vi "Insert.vi"(6 "Item":T1={"Item offset"=0, "Offset past Item"=0, "Name offset"=0, "Offset past Name"=0, "Found"=FALSE, "Item Type"=enum."Parser Error", "Item Index"=-1}, 9 "<JSON>name":string, 10 "JSON to Insert":string, 11 "JSON in":string) -> (1 "Inserted Item Offset":i32, 2 "Found":bool, 3 "string":string)   [LabVIEW 2017, in "JSONtext.lvlib"]
uses:
  JSONtext.lvlib
  Parsing/Found Items.ctl
  Parsing/Parsing State.ctl
  Parsing/Advance past whitespace.vi
  <vilib>/JDP Science/JDP Science Common Utilities/Trim Whitespace__JDP.vi
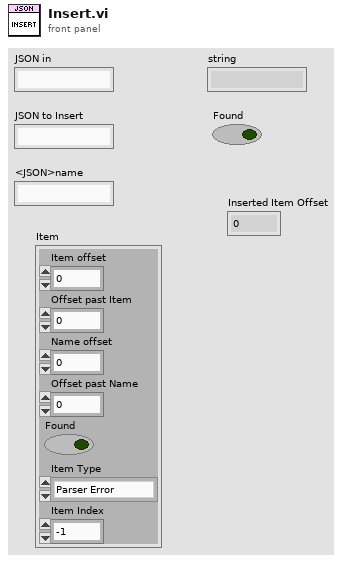
[diagram p1: front panel]
types:
  T1 = typedef "JSONtext.lvlib/Found Items.ctl" = cluster{"Item offset":i32, "Offset past Item":i32, "Name offset":i32, "Offset past Name":i32, "Found":bool, "Item Type":T2, "Item Index":i32}
  T2 = typedef "JSONtext.lvlib/Parsing State.ctl" = enum16{"Parser Error", "Object", "Array", "String", "Number/Other", "Leading Whitespace", "Object end", "Array end", "Value end"}
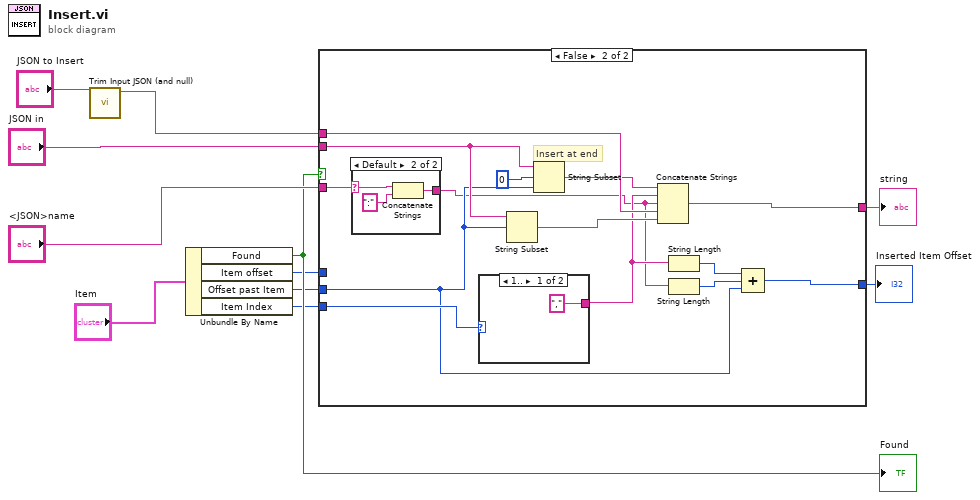
[diagram p0: block diagram]
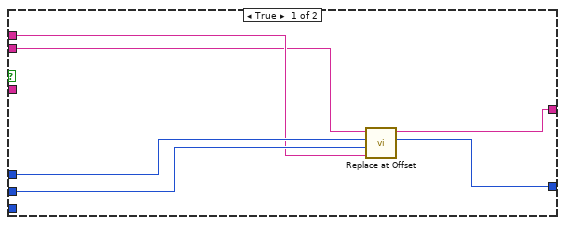
[diagram p2: hidden frame]
diagram:
  n1 = call "Trim Input JSON (and null).vi"("JSON Input"="JSON to Insert") -> ("<JSON>"=w1:string)  [unwired: 10 in]
  n2 = Unbundle By Name("Item") -> ("Found"=w10:bool, "Item offset"=w7:i32, "Offset past Item"=w6:i32, "Item Index"=w5:i32)
  "Found" <- w10
  n3 = case shown="False" w10 {
    tunnel: "JSON in" -> [w13 w31]
    tunnel: w1 -> [w14 w30]
    tunnel: [w17 w29] -> w8
    tunnel: "<JSON>name" -> [_ w19]
    tunnel: w7 -> [w16 _]
    tunnel: w6 -> [w15 w20]
    tunnel: w5 -> [_ w25]
    tunnel: [w12 w21] -> w3
    frame True {
      n4 = call "Replace at Offset.vi"("JSON to Insert"=w14, "Offset past Item"=w15, "Item offset"=w16, "<JSON> in"=w13) -> ("Item offset"=w12:i32, "<JSON>"=w17:string)  [unwired: 6 in]
    }
    frame False {
      # "Insert at end"
      n5 = case shown="Default" w19 {
        selector: w19 -> [_ w33]
        tunnel: [_ w32] -> w18
        frame "\u0000" {
          # "Array insert"
        }
        frame Default {
          n6 = Concatenate Strings(w33, ":" ("string")) -> (w32:string)
        }
      }
      n7 = case shown="1.." w25 {
        tunnel: ["," ("string") _] -> w24
        frame 1.. {
        }
        frame ..0 {
        }
      }
      n8 = String Subset(string=w31, offset (0)=w20) -> (substring=w26:string)  [unwired: 1 in]
      n9 = String Subset(string=w31, offset (0)=0 ("Value start in"), length (rest)=w20) -> (substring=w27:string)
      n10 = Concatenate Strings(w27, w24, w18, w30, w26) -> (w29:string)
      n11 = String Length(string=w24) -> (length=w23:i32)
      n12 = String Length(string=w18) -> (length=w22:i32)
      n13 = Compound Arithmetic op=ADD(w23, w22, w20) -> (w21:i32)
    }
  }
  "string" <- w8
  "Inserted Item Offset" <- w3
